vi "Terminate.vi"(8 "error in (no error)":errorcluster, 10 "Message in":refnum<class "TerminateMessage.lvclass">, 11 "Retiga in":refnum<class "Retiga.lvclass">) -> (0 "error out":errorcluster, 3 "Retiga out":refnum<class "Retiga.lvclass">)   [LabVIEW 2012, in "Retiga.lvclass"]
doc: "This member function is called when the statemachine in the run.vi receives an 'terminate' command. It closes the RabbitMQ connection. \n\nOverride this member function in your derived class to release all previously acquired resources (but don't forget to call the parent method). If your component has subcomponents, they count as resources, and you have to release them by calling their own terminate functions."
uses:
  Retiga.lvclass
  <vilib>/Distrio/Murmex/TerminateMessage/TerminateMessage.lvclass
  <vilib>/Distrio/Murmex/Murmex/Murmex.lvclass
panel:
  # "This method is called when the TERMINATE\ntrigger is sent. \n\nOverride this method when your component needs to\nrespond to this trigger. \n\nCall parent for proper implementation"
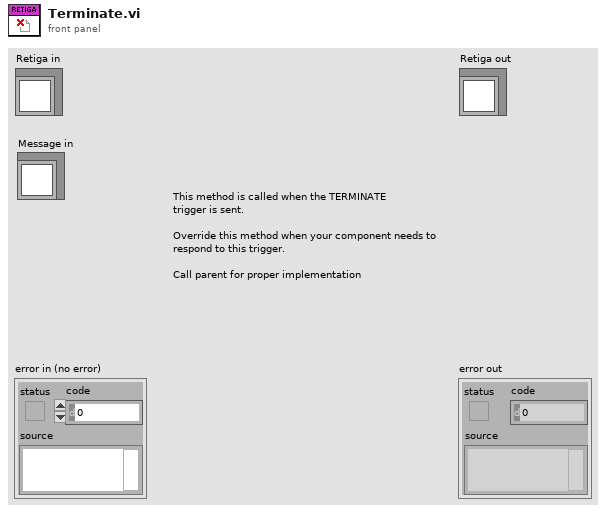
[diagram p1: front panel]
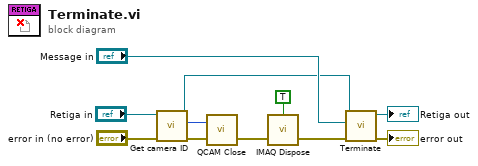
[diagram p0: block diagram]
diagram:
  n1 = call-dynamic "Get camera ID.vi"("error in (no error)"="error in (no error)", "Retiga in"="Retiga in") -> ("error out"=w5:errorcluster, "camera ID"=w4:u32, "Retiga out"=w6:refnum<class "Retiga.lvclass">)  [unwired: 7 in]
  n2 = call <userlib>:"QCAM Close.vi"("error in (no error)"=w5, "cameraId"=w4) -> ("error out"=w3:errorcluster)  [unwired: 1 in]
  n3 = call "IMAQ Dispose"("All Images? (No)"=TRUE, "error in (no error)"=w3) -> ("error out"=w2:errorcluster)  [unwired: 4 in]
  n4 = call-parent "Terminate.vi"("error in (no error)"=w2, "Message in"="Message in", "Murmex in"=w6) -> ("error out"=→"error out":errorcluster, "Murmex out"=→"Retiga out":refnum<class "Retiga.lvclass">)  [unwired: 7 in]
